vi "GetVersion.vi"() -> (3 "Version":string="9.9.9.9")   [LabVIEW 2021, in "ProligentXMLGenerator.lvlib" / "Datawarehouse.lvclass"]
uses:
  Datawarehouse.lvclass
  Datawarehouse.lvclass/Datawarehouse.ctl
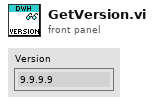
[diagram p1: front panel]
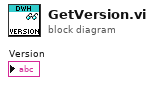
[diagram p0: block diagram]
diagram:
